vi "RGT Does File Exists.vi"(2 "error in (no error)":errorcluster, 3 "path":path) -> (0 "error out":errorcluster, 1 "file exists?":bool)   [LabVIEW 2020, in "NI_ReportGenerationCore.lvlib"]
uses:
  <vilib>/Utility/NIReport.llb/NI_ReportGenerationCore.lvlib
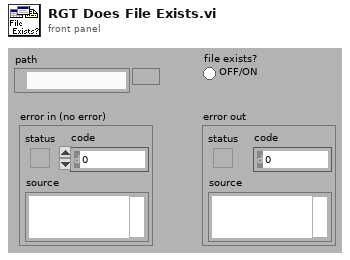
[diagram p1: front panel]
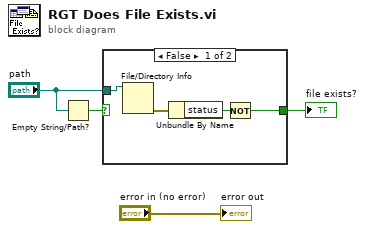
[diagram p0: block diagram]
diagram:
  n1 = Empty String/Path?(string/path="path") -> (empty?=w1:bool)
  n2 = case shown="False" w1 {
    tunnel: [w6 _] -> w3
    tunnel: "path" -> [w5 _]
    frame False {
      n3 = File/Directory Info(path=w5) -> (error out=w8:errorcluster)  [unwired: 1 in, 6 out]
      n4 = Unbundle By Name(w8) -> ("status"=w7:bool)
      n5 = Not(x=w7) -> (.not. x?=w6:bool)
    }
    frame True {
    }
  }
  "file exists?" <- w3
  "error out" <- "error in (no error)"
